vi "Destroy.vi"(0 "reference in":refnum<class "ZMQ_slave.lvclass">, 5 "error in (no error)":errorcluster) -> (14 "reference out":refnum<class "ZMQ_slave.lvclass">, 19 "error out":errorcluster)   [LabVIEW 2019, in "CommandResponse communication.lvlib" / "ZMQ_slave.lvclass"]
doc: "Destructor."
uses:
  ZMQ_slave.lvclass
  C:/Barkhausen mmWave radar/Development/LV/Barkhausen mmWave hardware control/Host/Intertarget communication/CR slave_class/CR slave.lvclass
  CR slave_class/CR slave.lvclass
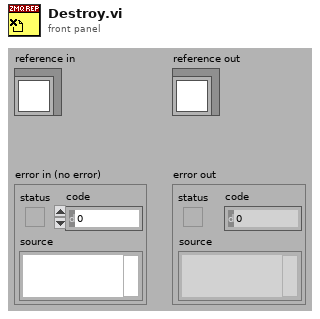
[diagram p1: front panel]
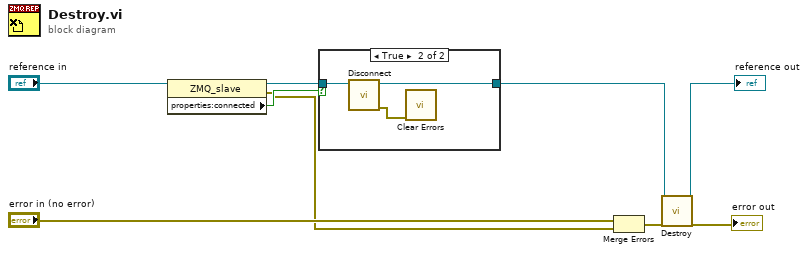
[diagram p0: block diagram]
diagram:
  n1 = property class="ZMQ_slave"(reference="reference in") -> (reference out=w4:refnum<class "ZMQ_slave.lvclass">, error out=w1:errorcluster, "properties:connected"=w2:bool)  [unwired: 1 in]
  n2 = case shown="True" w2 {
    tunnel: w4 -> [w10 w13]
    tunnel: [w10 w12] -> w3
    frame False {
    }
    frame True {
      n3 = call-dynamic "Disconnect.vi"("reference in"=w13) -> ("error out"=w11:errorcluster, "reference out"=w12:refnum<class "ZMQ_slave.lvclass">)  [unwired: 9 in]
      n4 = call <vilib>:"Clear Errors.vi"("error in (no error)"=w11) -> ()  [unwired: 5 in, 2 out]
    }
  }
  n5 = Merge Errors("error in (no error)", w1) -> (w8:errorcluster)
  n6 = call-parent "Destroy.vi"("reference in"=w3, "error in (no error)"=w8) -> ("reference out"=→"reference out":refnum<class "ZMQ_slave.lvclass">, "error out"=→"error out":errorcluster)  [unwired: 16 in]
